vi "Total Measured Energy.vi"(8 "error in (no error)":errorcluster, 10 "dt":dbl=2e-05 format="%#_13g", 11 "tdms file":refnum<k34>) -> (0 "error out":errorcluster, 2 "Total Test Energies (J)":dbl[](array[numeric]), 3 "tdms file out":refnum<k34>)   [LabVIEW 2015]
uses:
  <vilib>/Analysis/8numeric.llb/1D Numeric Integration.vi
  <vilib>/Analysis/NI_AALPro.lvlib
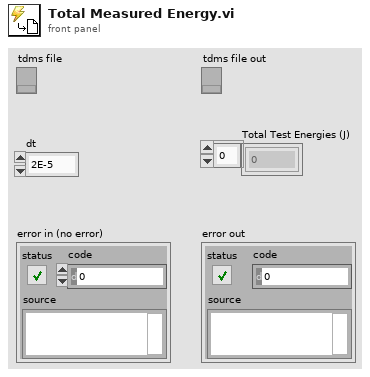
[diagram p1: front panel]
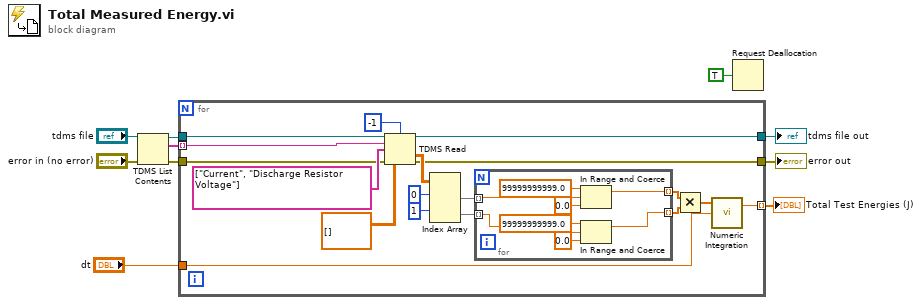
[diagram p0: block diagram]
diagram:
  n1 = TDMS List Contents(4:"error in (no error)", 7:"tdms file") -> (0:w5:errorcluster, 2:w4:string[], 3:w6:refnum<k34>)  [unwired: 1 in, 1 out]
  n2 = for {
    tunnel: w6 -> [w22]
    tunnel: [w13] -> w9
    tunnel: w5 -> [w21]
    tunnel: [w12] -> w10
    tunnel: w4 -> [w20] mode=indexing
    tunnel: [w19] -> w3 mode=indexing
    tunnel: "dt" -> [w11]
    n3 = TDMS Read(0:w22, 2:i64 -1 ("count (-1: all)"), 5:w20, 7:string[] ["Current", "Discharge Resistor Voltage"] ("channel name(s) in"), 11:w21, 12:dbl[][] []) -> (4:w13:refnum<k34>, 10:w18:dbl[][], 15:w12:errorcluster)  [unwired: 2 in, 3 out]
    n4 = Index Array(array=w18, index (row) #1=0 ("index (row)"), index (row) #2=1 ("index (row)")) -> (element #1=w17:dbl[], element #2=w16:dbl[])  [unwired: 2 in]
    n5 = for {
      tunnel: w17 -> [w36] mode=indexing
      tunnel: w16 -> [w32] mode=indexing
      tunnel: [w31] -> w15 mode=indexing
      tunnel: [w30] -> w14 mode=indexing
      n6 = In Range and Coerce(upper limit=99999999999.0, x=w36, lower limit=0.0) -> (coerced(x)=w31:dbl)  [unwired: 1 out]
      n7 = In Range and Coerce(upper limit=99999999999.0, x=w32, lower limit=0.0) -> (coerced(x)=w30:dbl)  [unwired: 1 out]
    }
    n8 = Multiply(x=w15, y=w14) -> (x*y=w28:dbl[])
    n9 = call-poly <vilib>:"Numeric Integration.vi"("dt"=w11, "Input Array"=w28) -> ("result"=w19:dbl)  [unwired: 1 in, 1 out]
  }
  "error out" <- w10
  "tdms file out" <- w9
  "Total Test Energies (J)" <- w3
  n10 = Request Deallocation(TRUE ("flag")) -> ()
